vi "GCMPlugin_GetInterfacePath.vi"(8 "error in (no error)":errorcluster, 11 "_BasicVIDocumentation in":refnum<class "ClassInheritanceEditor.lvclass">) -> (0 "error out":errorcluster, 2 "Path":path, 3 "_BasicVIDocumentation out":refnum<class "ClassInheritanceEditor.lvclass">)   [LabVIEW 2014, in "ClassInheritanceEditor.lvlib" / "ClassInheritanceEditor.lvclass"]
uses:
  ClassInheritanceEditor.lvclass
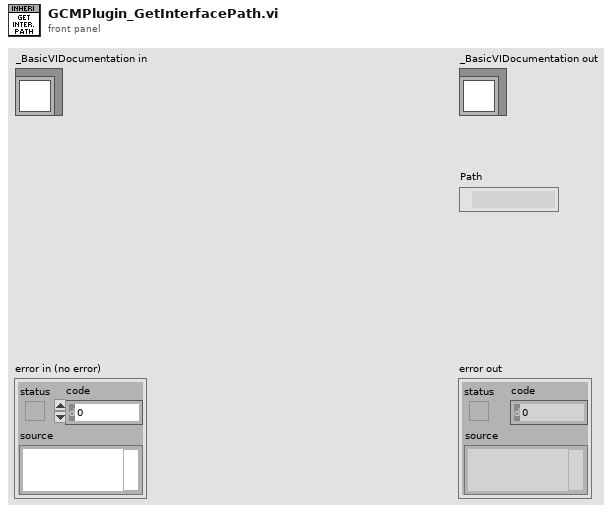
[diagram p1: front panel]
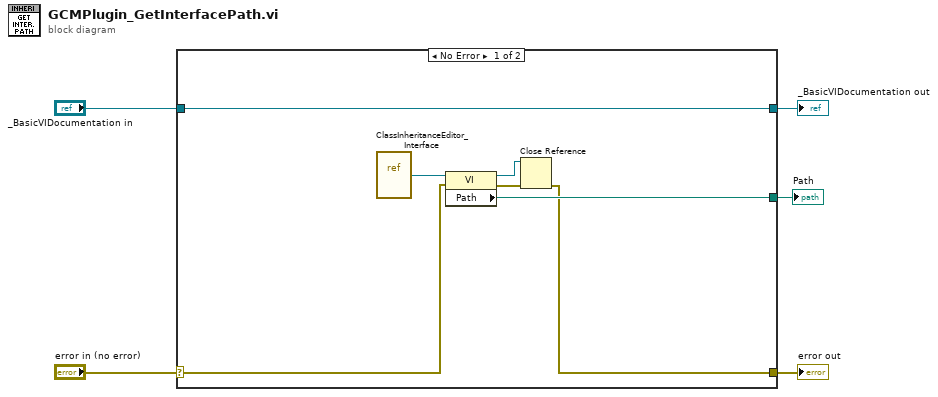
[diagram p0: block diagram]
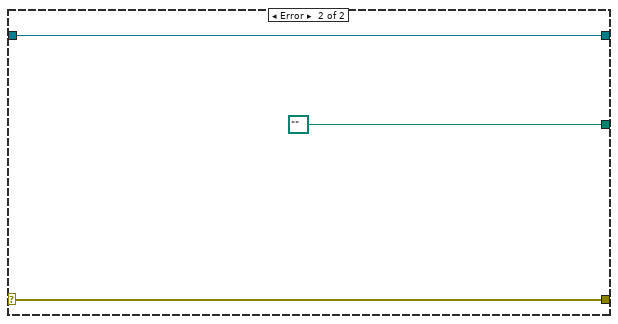
[diagram p2: hidden frame]
diagram:
  n1 = case shown="No Error" "error in (no error)" {
    selector: "error in (no error)" -> [w9 w15]
    tunnel: [w6 w15] -> w4
    tunnel: [w12 w14] -> w2
    tunnel: "_BasicVIDocumentation in" -> [w12 w14]
    tunnel: [w10 path "" ("Path")] -> w1
    frame No Error {
      n2 = vi-ref "ClassInheritanceEditor_Interface.vi"() -> (w11:refnum<vi>)
      n3 = property class="VI"(reference=w11, error in=w9) -> (reference out=w7:refnum<vi>, error out=w8:errorcluster, "Path"=w10:path)
      n4 = Close Reference(reference=w7, error in (no error)=w8) -> (error out=w6:errorcluster)
    }
    frame Error {
    }
  }
  "error out" <- w4
  "_BasicVIDocumentation out" <- w2
  "Path" <- w1
